vi "CreateWO-CheckRequiredFields.vi"(8 "error in (no error)":errorcluster, 11 "ERP-CreateWorkOrder in":refnum<class "ERP-CreateWorkOrder.lvclass">) -> (0 "error out":errorcluster, 2 "Create Work Order":bool, 3 "ERP-CreateWorkOrder out":refnum<class "ERP-CreateWorkOrder.lvclass">)   [LabVIEW 2013, in "ERP-CreateWorkOrder.lvclass"]
uses:
  ERP-CreateWorkOrder.lvclass
  ERP-CreateWorkOrder.lvclass/ERP-CreateWorkOrder.ctl
  <userlib>/_OpenG.lib/array/array.llb/Search 1D Array (Boolean)__ogtk.vi
  <userlib>/_OpenG.lib/array/array.llb/Empty 1D Array (I32)__ogtk.vi
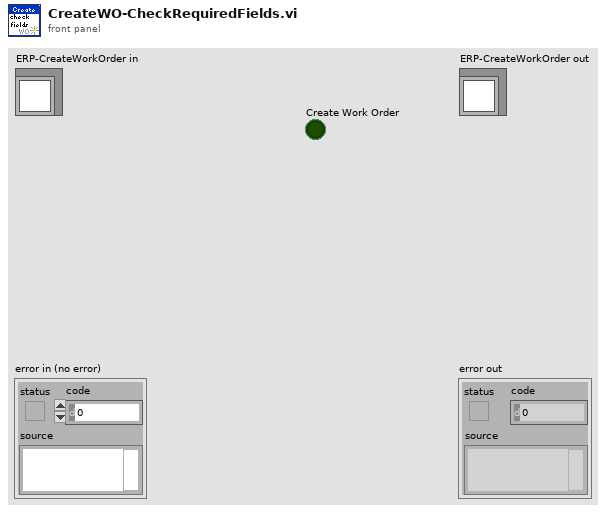
[diagram p1: front panel]
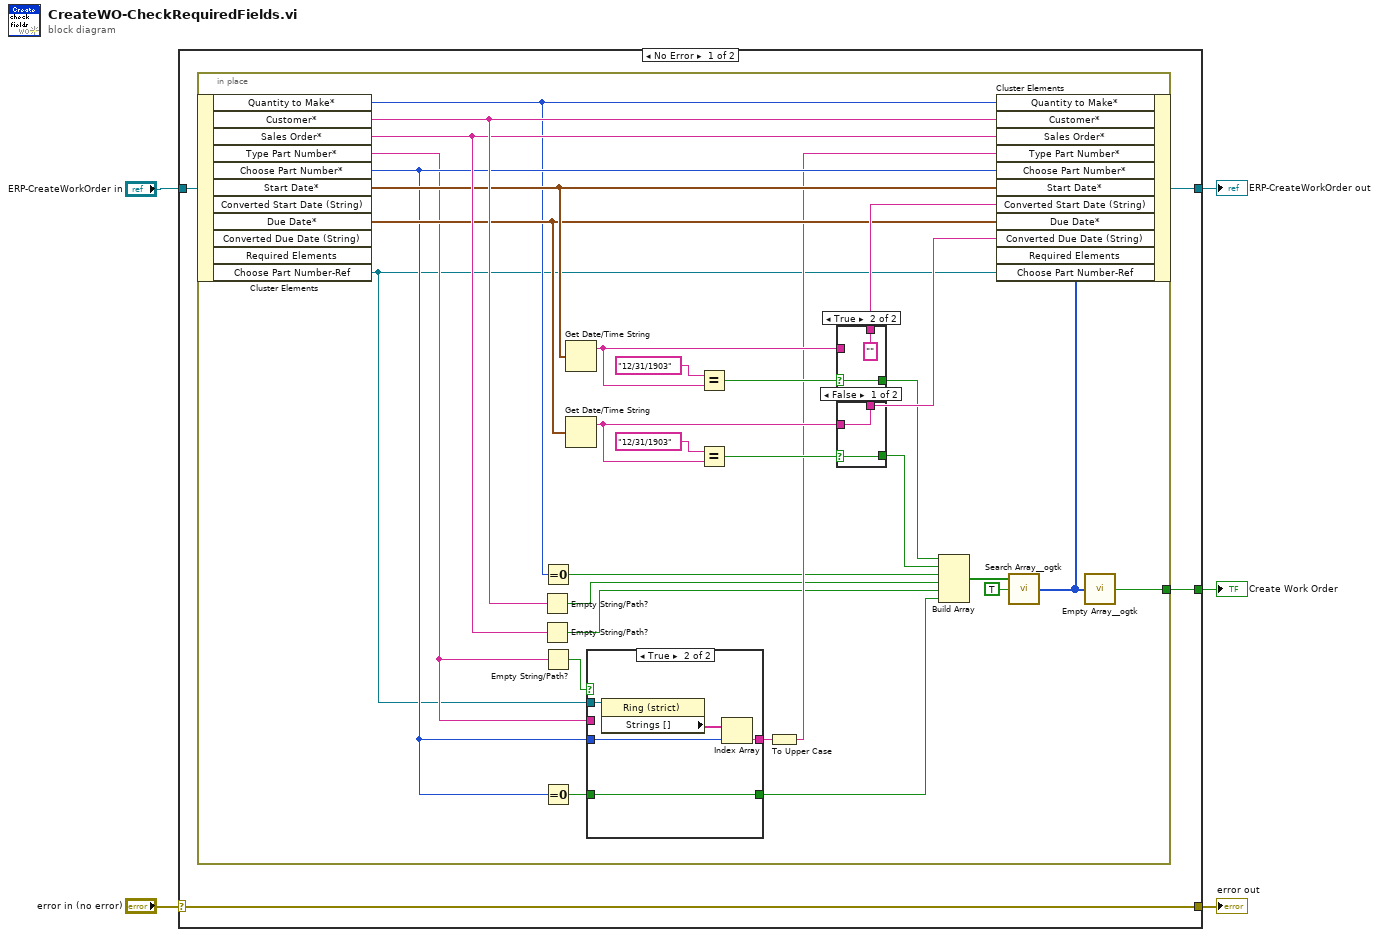
[diagram p0: block diagram]
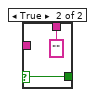
[diagram p3: hidden frame]
diagram:
  n1 = case shown="No Error" "error in (no error)" {
    selector: "error in (no error)" -> [w9 w56]
    tunnel: [w9 w56] -> w4
    tunnel: [w7 w55] -> w2
    tunnel: "ERP-CreateWorkOrder in" -> [w8 w55]
    tunnel: [w6 _] -> w1
    frame No Error {
      n2 = in-place {
        in-place-border: [w13] -> w6
        n3 = in-place-cluster #1(w8) -> ("Quantity to Make*"=w22:i32, "Customer*"=w39:string, "Sales Order*"=w38:string, "Type Part Number*"=w25:string, "Choose Part Number*"=w26:u16, "Start Date*"=w37:timestamp, "Due Date*"=w31:timestamp, "Choose Part Number-Ref"=w10:refnum<vi>)  [unwired: 3 out]
        n4 = Empty String/Path?(string/path=w39) -> (empty?=w16:bool)
        n5 = Empty String/Path?(string/path=w38) -> (empty?=w15:bool)
        n6 = Equal To 0?(x=w22) -> (x = 0?=w17:bool)
        n7 = Empty String/Path?(string/path=w25) -> (empty?=w27:bool)
        n8 = Equal To 0?(x=w26) -> (x = 0?=w21:bool)
        n9 = Get Date/Time String(seconds (now)=w37) -> (date string=w35:string)  [unwired: 2 in, 1 out]
        n10 = Get Date/Time String(seconds (now)=w31) -> (date string=w33:string)  [unwired: 2 in, 1 out]
        n11 = case shown="True" w27 {
          selector: w27 -> [w40 _]
          tunnel: w10 -> [_ w46]
          tunnel: w26 -> [_ w44]
          tunnel: [w41 w43] -> w24
          tunnel: w25 -> [w41 _]
          tunnel: [w40 w42] -> w14
          tunnel: w21 -> [_ w42]
          frame False {
          }
          frame True {
            n12 = property class="Ring (strict)"(reference=w46) -> ("Strings []"=w45:string[])  [unwired: 1 in, 2 out]
            n13 = Index Array(array=w45, index=w44) -> (element=w43:string)
          }
        }
        n14 = Equal?(x="12/31/1903", y=w35) -> (x = y?=w29:bool)
        n15 = Equal?(x="12/31/1903", y=w33) -> (x = y?=w28:bool)
        n16 = To Upper Case(1:w24) -> (0:w23:string)
        n17 = case shown="True" w29 {
          selector: w29 -> [w51 w53]
          tunnel: w35 -> [w52 _]
          tunnel: [w52 "" ("date string")] -> w34
          tunnel: [w51 w53] -> w19
          frame False {
          }
          frame True {
          }
        }
        n18 = case shown="False" w28 {
          selector: w28 -> [w47 w49]
          tunnel: w33 -> [w48 _]
          tunnel: [w48 "" ("date string")] -> w30
          tunnel: [w47 w49] -> w18
          frame False {
          }
          frame True {
          }
        }
        n19 = Build Array(w19, w18, w17, w16, w15, w14) -> (w20:bool[])
        n20 = call-poly <userlib>:"Search Array__ogtk.vi"("Array"=w20, "Element Data"=TRUE) -> ("Indices of Elements"=w11:i32[])  [unwired: 7 in]
        n21 = in-place-cluster #1("Quantity to Make*"=w22, "Customer*"=w39, "Sales Order*"=w38, "Type Part Number*"=w23, "Choose Part Number*"=w26, "Start Date*"=w37, "Converted Start Date (String)"=w34, "Due Date*"=w31, "Converted Due Date (String)"=w30, "Required Elements"=w11, "Choose Part Number-Ref"=w10) -> (w7:refnum<class "ERP-CreateWorkOrder.lvclass">)
        n22 = call-poly <userlib>:"Empty Array__ogtk.vi"("Array"=w11) -> ("Empty Array?"=w13:bool)  [unwired: 8 in]
      }
    }
    frame Error {
    }
  }
  "error out" <- w4
  "ERP-CreateWorkOrder out" <- w2
  "Create Work Order" <- w1
